vi "Waveform Shift.vi"(8 "Input Data Valid":bool, 10 "Acquisition Status In":T1={"Reset"=FALSE, "Acquisition Engine Start (Arm)"=FALSE, "Current State"=enum."Acquire Pre-Trigger Samples", "Trig Offset"=0, "Points Unread"=0, "Points Acquired"=0, "Records Done"=0, "Start of Read"=FALSE, "End of Read"=FALSE, "Start of Record"=FALSE, "End of Record"=FALSE, "Ready for Ref Trig"=FALSE, "In Reset?"=FALSE}, 11 "Input Data":i16[](array[numeric])=[0, 0, 0, 0]) -> (0 "Output Data Valid":bool, 2 "Acquisition StatusOut":T1={"Reset"=FALSE, "Acquisition Engine Start (Arm)"=FALSE, "Current State"=enum."Acquire Pre-Trigger Samples", "Trig Offset"=0, "Points Unread"=0, "Points Acquired"=0, "Records Done"=0, "Start of Read"=FALSE, "End of Read"=FALSE, "Start of Record"=FALSE, "End of Record"=FALSE, "Ready for Ref Trig"=FALSE, "In Reset?"=FALSE}, 3 "Output Data":i16[](array[numeric]))   [LabVIEW 2012]
uses:
  Acquisition Engine/Acquisition Status.ctl
  Acquisition Engine/Acquisition Engine State.ctl
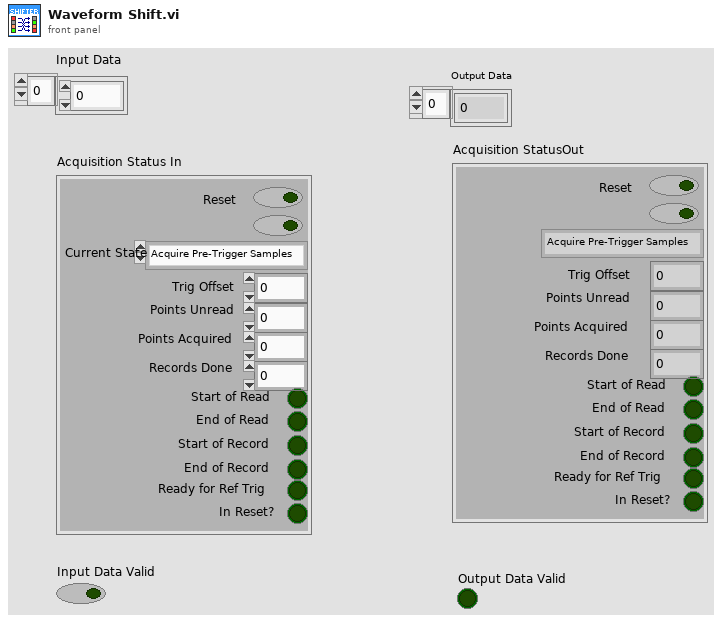
[diagram p1: front panel]
types:
  T1 = typedef "Acquisition Status.ctl" = cluster{"Reset":bool, "Acquisition Engine Start (Arm)":bool, "Current State":T2, "Trig Offset":u8, "Points Unread":u16, "Points Acquired":u16, "Records Done":u16, "Start of Read":bool, "End of Read":bool, "Start of Record":bool, "End of Record":bool, "Ready for Ref Trig":bool, "In Reset?":bool}
  T2 = typedef "Acquisition Engine State.ctl" = enum8{"Idle", "Arm Acquisition Engine", "Acquire Pre-Trigger Samples", "Wait for Trigger", "Acquisition Hold Off Time", "Read Data from Buffer", "Check Records Done?", "Re-Arm State", "Flush Available Data"}
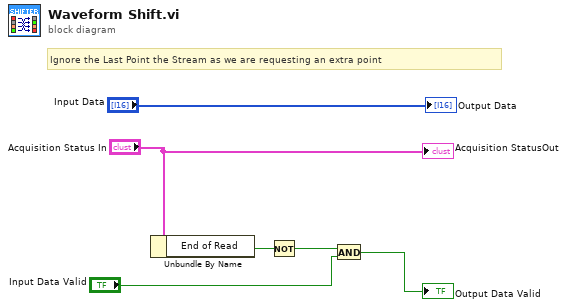
[diagram p0: block diagram]
diagram:
  # "Ignore the Last Point the Stream as we are requesting an extra point"
  n1 = Unbundle By Name("Acquisition Status In") -> ("End of Read"=w4:bool)
  n2 = Not(x=w4) -> (.not. x?=w3:bool)
  n3 = And(x=w3, y="Input Data Valid") -> (x .and. y?=→"Output Data Valid":bool)
  "Acquisition StatusOut" <- "Acquisition Status In"
  "Output Data" <- "Input Data"
